vi "Instrument Get By ixInstrument.vi"(8 "error in (no error)":errorcluster, 10 "ixInstrument":i32, 11 "Connection Refnum":T1) -> (0 "error out":errorcluster, 2 "Instrument Record":T2, 3 "Connection Refnum":T1, 4 "Data Present?":bool)   [LabVIEW 2011]
uses:
  Instrument Record.ctl
  Summitek EXT/ODBC/SQL Controls/Connection Refnum.ctl
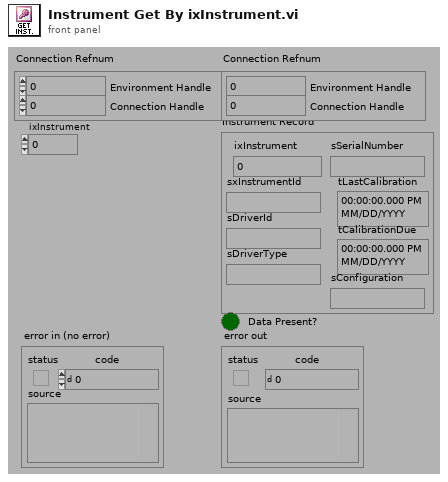
[diagram p1: front panel]
types:
  T1 = typedef "Connection Refnum.ctl" = cluster{"Environment Handle":i32, "Connection Handle":i32}
  T2 = typedef "Instrument Record.ctl" = cluster{"ixInstrument":i32, "sxInstrumentId":string, "sDriverId":string, "sDriverType":string, "sSerialNumber":string, "tLastCalibration":timestamp, "tCalibrationDue":timestamp, "sConfiguration":string}
  T3 = typedef "Statement Refnum.ctl" = cluster{"Statement Handle":i32, "Parameter Number":u16}
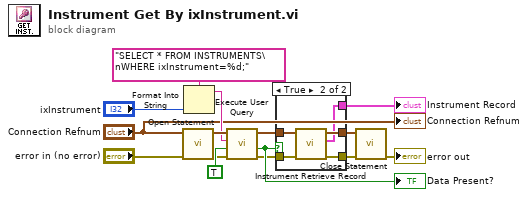
[diagram p0: block diagram]
diagram:
  n1 = call "Open Statement.vi"("error in (no error)"="error in (no error)", "Connection Refnum"="Connection Refnum") -> ("error out"=w10:errorcluster, "Statement Refnum"=w11:T3)  [unwired: 4 out]
  n2 = Format Into String(format string="SELECT * FROM INSTRUMENTS\nWHERE ixInstrument=%d;" ("Query Name"), "ixInstrument") -> (resulting string=w7:string)  [unwired: 2 in, 1 out]
  n3 = call "Execute User Query.vi"("error in (no error)"=w10, "Return Data? (f)"=TRUE, "User Query"=w7, "Statement Refnum"=w11) -> ("error out"=w14:errorcluster, "Data Present?"=w15:bool, "Statement Refnum"=w13:T3)  [unwired: 1 out]
  "Data Present?" <- w15
  n4 = case shown="True" w15 {
    tunnel: w14 -> [w16 w22]
    tunnel: w13 -> [w17 w21]
    tunnel: [w16 w19] -> w9
    tunnel: [w17 w20] -> w8
    tunnel: [_ w18] -> w3
    frame False {
    }
    frame True {
      n5 = call "Instrument Retrieve Record.vi"("error in (no error)"=w22, "Statement Refnum"=w21) -> ("error out"=w19:errorcluster, "Instrument"=w18:T2, "Statement Refnum"=w20:T3)  [unwired: 7 out]
    }
  }
  "Instrument Record" <- w3
  n6 = call "Close Statement.vi"("error in (no error)"=w9, "Statement Refnum"=w8) -> ("error out"=→"error out":errorcluster)  [unwired: 5 out]
  "Connection Refnum" <- "Connection Refnum"
